vi "RT Main_Simple.vi"() -> ()   [LabVIEW 2015]
uses:
  <vilib>/NI/cRIO Wfm/cRIO Wfm.lvlib
  <vilib>/NI/cRIO Wfm/AcqRead(Wfm).vi
  <vilib>/rvi/interface/nirviOpenFPGA/nirviOpenFPGA.xnode
  <vilib>/rvi/interface/nirviMethod/nirviMethod.xnode
  <vilib>/FPGAPlugInAG/Dynamic/niLvFpga_Reset_Dynamic.vi
  <vilib>/FPGAPlugInAG/Dynamic/niLvFpga_Run_Dynamic.vi
  <vilib>/rvi/interface/nirviCloseFPGA/nirviCloseFPGA.xnode
  <vilib>/FPGAPlugInAG/Dynamic/niLvFpga_Close_Dynamic.vi
  <vilib>/NI/cRIO Wfm/ChannelConfig.ctl
  FPGA Bitfiles/SOMHands-On_FPGATarget_FPGAMainSPIAPIwi_bu6rYlCdJlM.lvbitx
  FPGA Main_SPI API with Waveform Library.vi
  <vilib>/FPGAPlugInAG/sbRIO-9651/niLvFpga_Open_sbRIO-9651.vi
  <vilib>/rvi/interface/common/dynamic/niFpgaDynamicAddResources.vi
panel:
  out "Waveform Graph":waveform(sgl)[](graph)
  in  "scan rate [S/s]":u32=25000
  in  "quit":bool
  in  "number of samples":i32=2000 min=128
  in  "Samples per Channel":i32=1000
  # "Channel Settings"
  # "VI Controls"
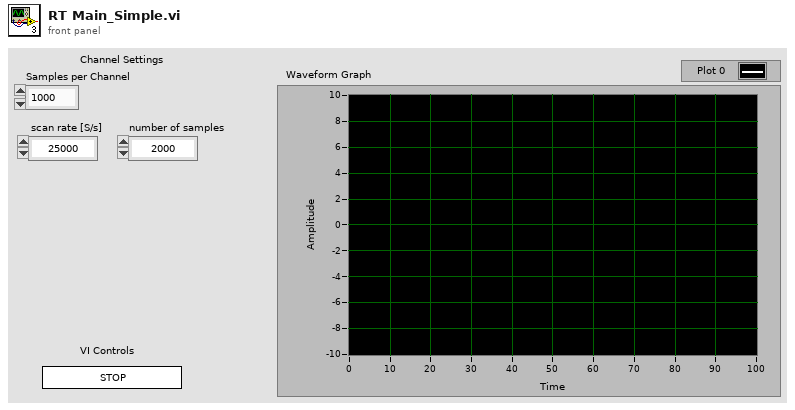
[diagram p1: front panel]
types:
  T1 = typedef "cRIO Wfm.lvlib/ChannelConfig.ctl" = cluster{"Channel Name":string, "Sensitivity mV_EU":dbl, "EU":string, "dB Ref EU":dbl}[]
  T2 = typedef "cRIO Wfm.lvlib/SamplingInfo.ctl" = cluster{"Number of Channels":i32, "Actual Samp Rate":dbl, "Chan Name Array":string[], "EU Chan Array":string[], "dB Ref Chan Array":dbl[]}
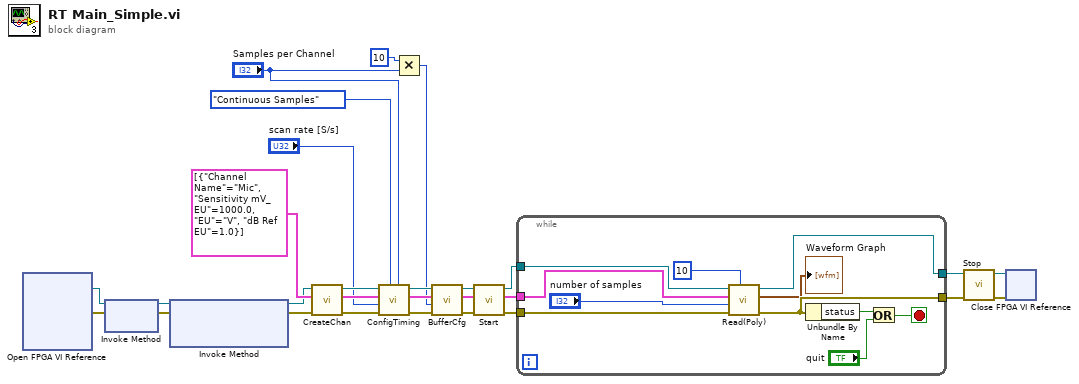
[diagram p0: block diagram]
diagram:
  n1 = xnode "Open FPGA VI Reference"() -> ("FPGA VI Reference Out"=w14:refnum<k20>, "error out"=w15:errorcluster)  [unwired: 2 in]
  n2 = xnode "Invoke Method"("FPGA VI Reference In"=w14, "error in"=w15) -> ("FPGA VI Reference Out"=w13:refnum<k20>, "error out"=w10:errorcluster)
  n3 = xnode "Invoke Method"("FPGA VI Reference In"=w13, "error in"=w10) -> ("FPGA VI Reference Out"=w12:refnum<k20>, "error out"=w11:errorcluster)  [unwired: 1 in]
  n4 = call <vilib>:"CreateChan.vi"("error in"=w11, "Channel Info"=T1 [{"Channel Name"="Mic", "Sensitivity mV_EU"=1000.0, "EU"="V", "dB Ref EU"=1.0}], "Dynamic FPGA Ref"=w12) -> ("error out"=w18:errorcluster, "Sampling Info"=w22:T2, "Dynamic FPGA Ref Out"=w28:refnum<k20>)  [unwired: 6 in]
  n5 = call <vilib>:"ConfigTiming.vi"("Samples per Channel"="Samples per Channel", "Sample Mode"=enum16{"Finite Samples", "Continuous Samples"}."Continuous Samples", "error in"=w18, "Sample Rate"="scan rate [S/s]", "Sampling Info In"=w22, "Dynamic FPGA Ref"=w28) -> ("error out"=w17:errorcluster, "Sampling Info Out"=w23:T2, "Dynamic FPGA Ref Out"=w27:refnum<k20>)  [unwired: 2 in, 1 out]
  n6 = Multiply(x=10, y="Samples per Channel") -> (x*y=w19:i32)
  n7 = call <vilib>:"BufferCfg.vi"("error in"=w17, "Buffer Size [Samps per Chan]"=w19, "Sampling Info In"=w23, "Dynamic FPGA Ref"=w27) -> ("error out"=w16:errorcluster, "Sampling Info Out"=w21:T2, "Dynamic FPGA Ref Out"=w26:refnum<k20>)  [unwired: 4 in, 1 out]
  n8 = call <vilib>:"Start.vi"("error in"=w16, "Sampling Info In"=w21, "Dynamic FPGA Ref"=w26) -> ("error out"=w2:errorcluster, "Sampling Info Out"=w1:T2, "Dynamic FPGA Ref Out"=w3:refnum<k20>)  [unwired: 6 in]
  n9 = while {
    tunnel: [w33] -> w5
    tunnel: [w36] -> w6
    tunnel: w3 -> [w35]
    tunnel: w2 -> [w32]
    tunnel: w1 -> [w30]
    stop <- w38 stop-if-true
    n10 = call-poly <vilib>:"Read(Poly).vi"("Poll Time (ms)"=u32 10, "error in"=w32, "Samps Read per Chan"="number of samples", "Sampling Info"=w30, "Dynamic FPGA Ref"=w35) -> ("error out"=w33:errorcluster, "Wfm Data"=→"Waveform Graph":waveform(sgl)[], "Dynamic FPGA Ref Out"=w36:refnum<k20>)  [unwired: 3 in, 1 out]
    n11 = Unbundle By Name(w33) -> ("status"=w37:bool)
    n12 = Or(x=w37, y="quit") -> (x .or. y?=w38:bool)
  }
  n13 = call <vilib>:"Stop.vi"("error in"=w5, "Dynamic FPGA Ref"=w6) -> ("error out"=w8:errorcluster, "Dynamic FPGA Ref Out"=w9:refnum<k20>)  [unwired: 8 in]
  n14 = xnode "Close FPGA VI Reference"("FPGA VI Reference In"=w9, "error in"=w8) -> ()  [unwired: 1 out]
